vi "Test VI.vi"() -> ()   [LabVIEW 2020]
uses:
  MulColLBTable/MulColLBTable/MulColLBTable.lvclass
  <vilib>/Utility/miscctls.llb/LVRowAndColumnTypeDef.ctl
panel:
  out "Selected Cell":T1
  out "error out 2":errorcluster
  in  "Multicolumn Listbox 2":i32(listbox)
  out "error out":errorcluster
  in  "stop":bool
  in  "Multicolumn Listbox":i32[](listbox)
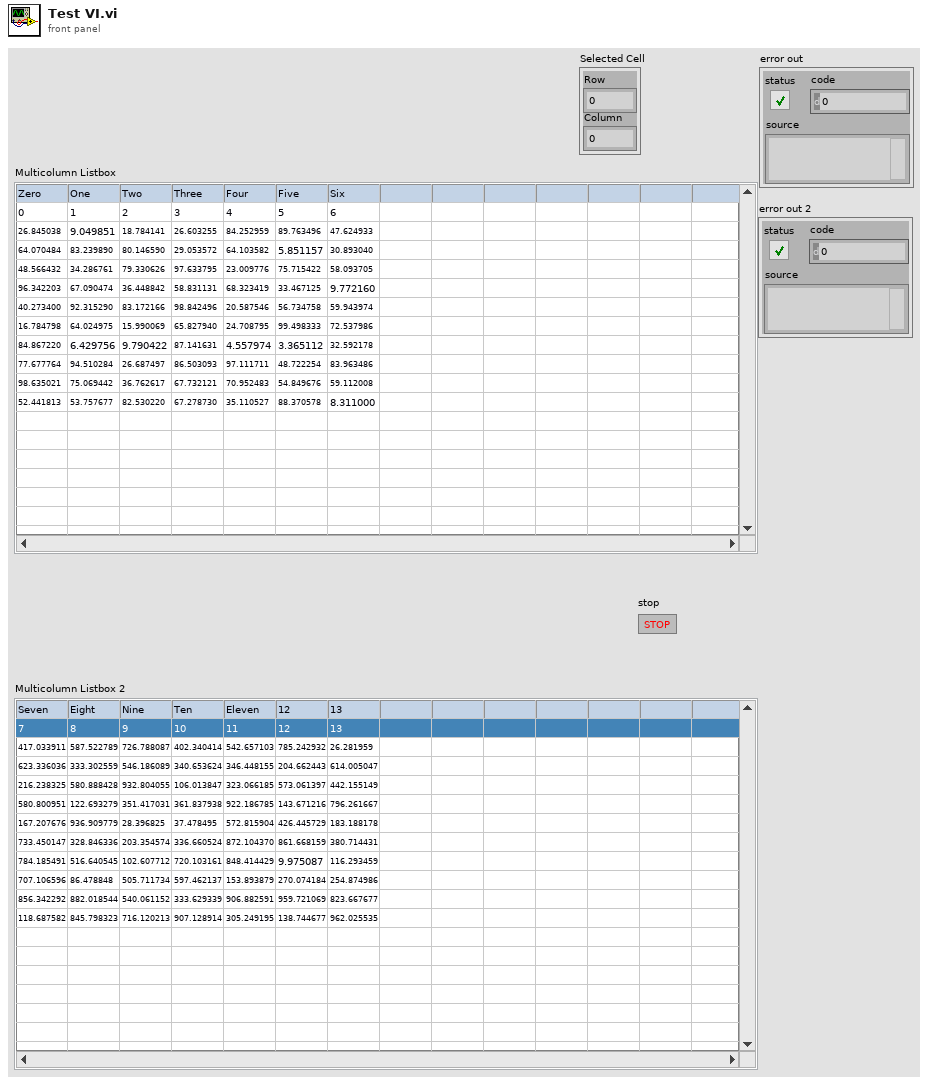
[diagram p1: front panel]
types:
  T1 = typedef "LVRowAndColumnTypeDef.ctl" = cluster{"Row":i32, "Column":i32}
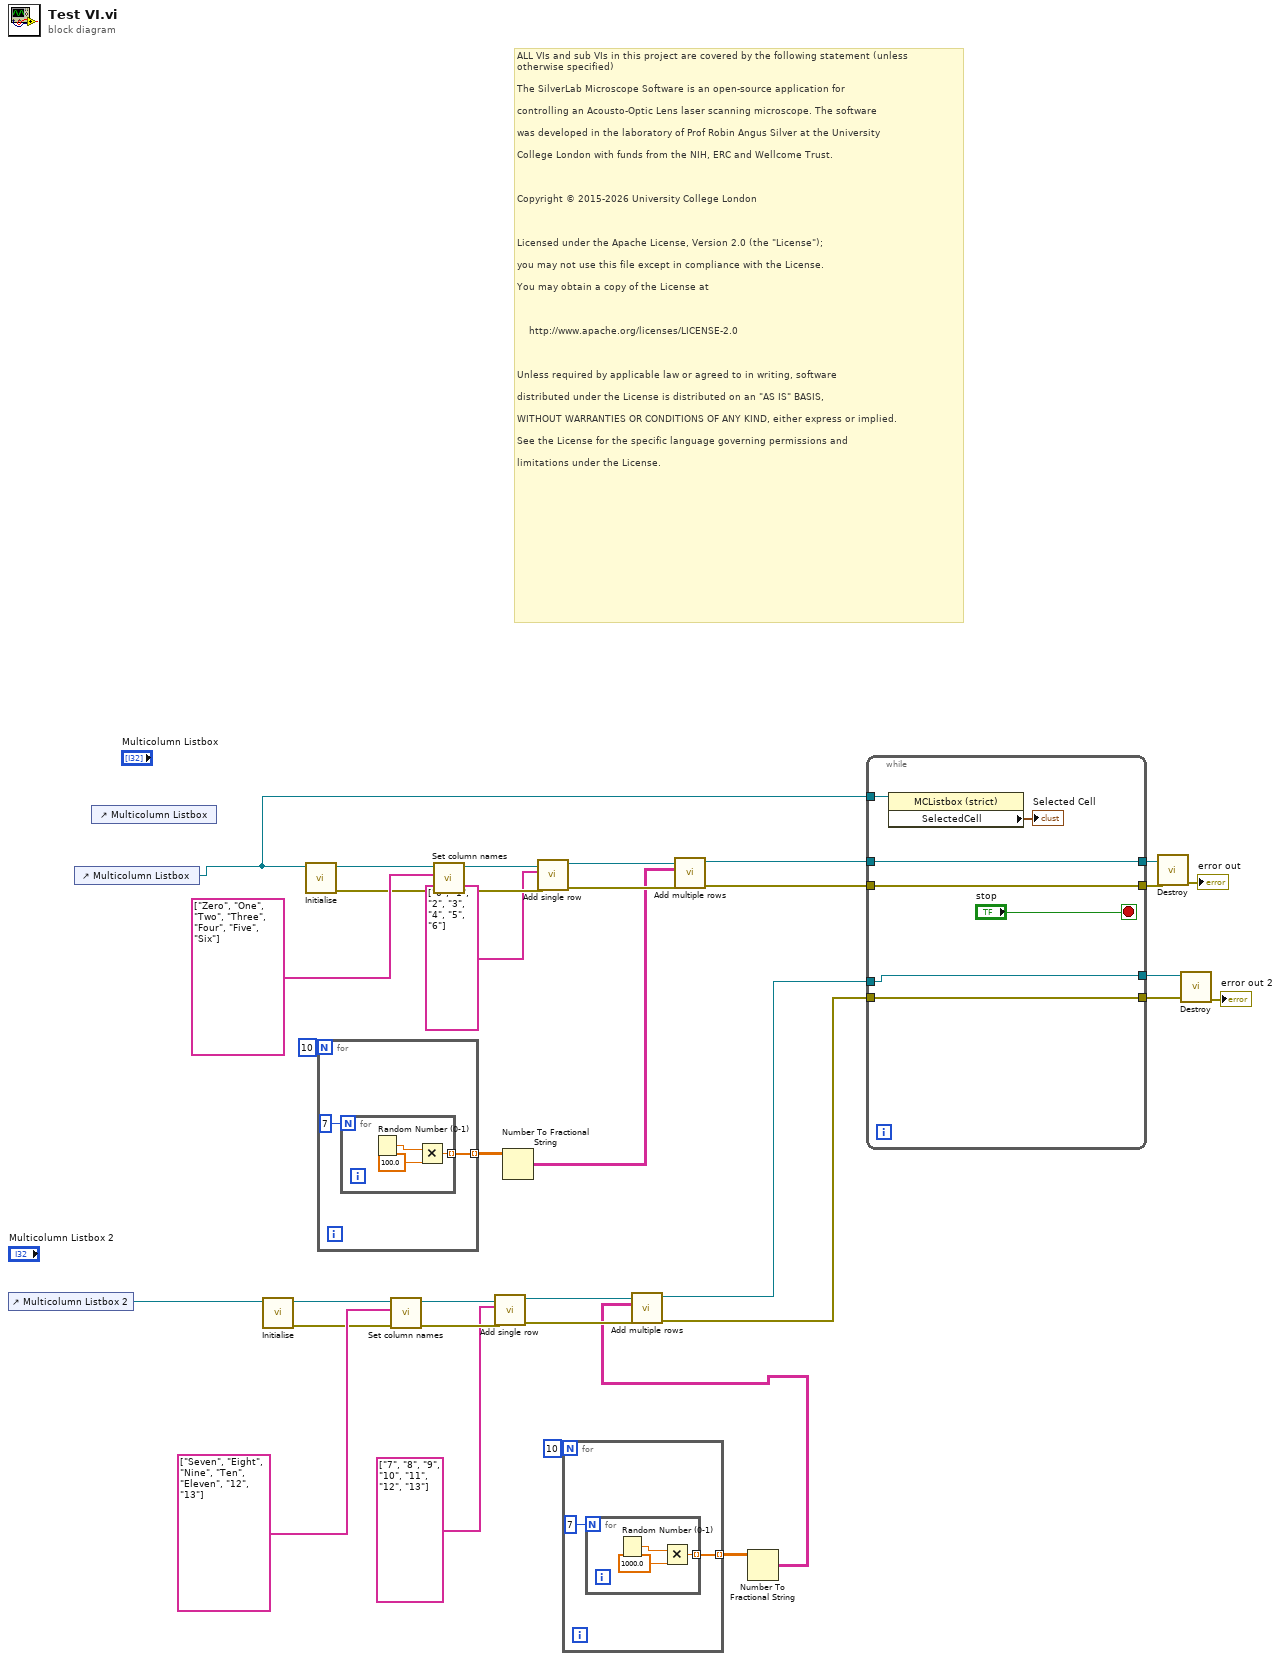
[diagram p0: block diagram]
diagram:
  # "ALL VIs and sub VIs in this project are covered by the following statement (unless \notherwise specified)\n\nThe SilverLab Microscope Software is an open-source application for\n\ncontrolling an Acousto-Optic Lens laser scanning microscope. The software\n\nwas developed in the laboratory of Prof Robin Angus Silver at the University\n\nCollege London with funds from the NIH, ERC and Wellcome Trust.\n\n \n\nCopyright © 2015-2026 University College London\n\n \n\nLicensed under the Apache License, Version 2.0 (the \"License\");\n\nyou may not use this file except in compliance with the License.\n\nYou may obtain a copy of the License at\n\n \n\n    http://www.apache.org/licenses/LICENSE-2.0\n\n \n\nUnless required by applicable law or agreed to in writing, software\n\ndistributed under the License is distributed on an \"AS IS\" BASIS,\n\nWITHOUT WARRANTIES OR CONDITIONS OF ANY KIND, either express or implied.\n\nSee the License for the specific language governing permissions and\n\nlimitations under the License."
  n1 = control-ref of="Multicolumn Listbox 2"() -> (w8:refnum<vi>)
  n2 = control-ref of="Multicolumn Listbox"() -> (w2:refnum<vi>)
  n3 = control-ref of="Multicolumn Listbox"() -> (w1:refnum<vi>)
  n4 = call "Initialise.vi"("Multicolumn Listbox"=w8) -> ("error out"=w17:errorcluster, "MulColLBTable.lvclass out"=w19:refnum<class "MulColLBTable.lvclass">)  [unwired: 9 in]
  n5 = call "Initialise.vi"("Multicolumn Listbox"=w2) -> ("error out"=w33:errorcluster, "MulColLBTable.lvclass out"=w35:refnum<class "MulColLBTable.lvclass">)  [unwired: 9 in]
  n6 = for {
    N: 10 -> [_]
    tunnel: [w37] -> w29 mode=indexing
    n7 = for {
      N: 7 -> [_]
      tunnel: [w38] -> w37 mode=indexing
      n8 = Random Number (0-1)() -> (number: 0 to 1=w40:dbl)
      n9 = Multiply(x=w40, y=100.0) -> (x*y=w38:dbl)
    }
  }
  n10 = call "Set column names.vi"("error in (no error)"=w17, "Column Header Strings[]"=string[] ["Seven", "Eight", "Nine", "Ten", "Eleven", "12", "13"], "MulColLBTable.lvclass"=w19) -> ("error out"=w16:errorcluster, "MulColLBTable.lvclass 2"=w15:refnum<class "MulColLBTable.lvclass">)  [unwired: 7 in]
  n11 = call "Set column names.vi"("error in (no error)"=w33, "Column Header Strings[]"=string[] ["Zero", "One", "Two", "Three", "Four", "Five", "Six"], "MulColLBTable.lvclass"=w35) -> ("error out"=w32:errorcluster, "MulColLBTable.lvclass 2"=w31:refnum<class "MulColLBTable.lvclass">)  [unwired: 7 in]
  n12 = call "Add single row.vi"("error in (no error)"=w16, "Row"=string[] ["7", "8", "9", "10", "11", "12", "13"], "MulColLBTable.lvclass"=w15) -> ("error out"=w11:errorcluster, "MulColLBTable.lvclass 2"=w10:refnum<class "MulColLBTable.lvclass">)  [unwired: 7 in]
  n13 = Number To Fractional String(number=w29) -> (F-format string=w25:string[][])  [unwired: 3 in]
  n14 = call "Add single row.vi"("error in (no error)"=w32, "Row"=string[] ["0", "1", "2", "3", "4", "5", "6"], "MulColLBTable.lvclass"=w31) -> ("error out"=w27:errorcluster, "MulColLBTable.lvclass 2"=w26:refnum<class "MulColLBTable.lvclass">)  [unwired: 7 in]
  n15 = for {
    N: 10 -> [_]
    tunnel: [w42] -> w13 mode=indexing
    n16 = for {
      N: 7 -> [_]
      tunnel: [w43] -> w42 mode=indexing
      n17 = Random Number (0-1)() -> (number: 0 to 1=w45:dbl)
      n18 = Multiply(x=w45, y=1000.0) -> (x*y=w43:dbl)
    }
  }
  n19 = call "Add multiple rows.vi"("error in (no error)"=w27, "Row"=w25, "MulColLBTable.lvclass"=w26) -> ("error out"=w24:errorcluster, "MulColLBTable.lvclass 2"=w23:refnum<class "MulColLBTable.lvclass">)  [unwired: 7 in]
  n20 = Number To Fractional String(number=w13) -> (F-format string=w9:string[][])  [unwired: 3 in]
  n21 = call "Add multiple rows.vi"("error in (no error)"=w11, "Row"=w9, "MulColLBTable.lvclass"=w10) -> ("error out"=w5:errorcluster, "MulColLBTable.lvclass 2"=w7:refnum<class "MulColLBTable.lvclass">)  [unwired: 7 in]
  n22 = while {
    tunnel: w24 -> [w50]
    tunnel: w23 -> [w51]
    tunnel: [w51] -> w22
    tunnel: [w50] -> w21
    tunnel: w7 -> [w49]
    tunnel: [w49] -> w6
    tunnel: w5 -> [w48]
    tunnel: [w48] -> w4
    tunnel: w2 -> [w47]
    stop <- "stop" stop-if-true
    n23 = property class="MCListbox (strict)"(reference=w47) -> ("SelectedCell"=→"Selected Cell":T1)  [unwired: 1 in, 2 out]
  }
  n24 = call "Destroy.vi"("error in (no error)"=w21, "MulColLBTable.lvclass"=w22) -> ("error out"=→"error out":errorcluster)  [unwired: 9 in]
  n25 = call "Destroy.vi"("error in (no error)"=w4, "MulColLBTable.lvclass"=w6) -> ("error out"=→"error out 2":errorcluster)  [unwired: 9 in]
